vi "SegmentAndCircleIntersection.vi"(8 "CircleRadius":dbl, 9 "CircleCenter":dbl[](array[numeric]), 10 "SegmentPointB":dbl[](array[numeric]), 11 "SegmentPointA":dbl[](array[numeric])) -> (1 "DoTheyIntersect?":bool)   [LabVIEW 2017]
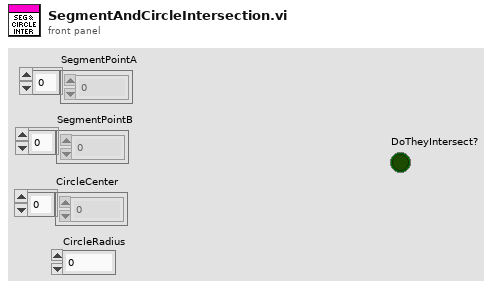
[diagram p1: front panel]
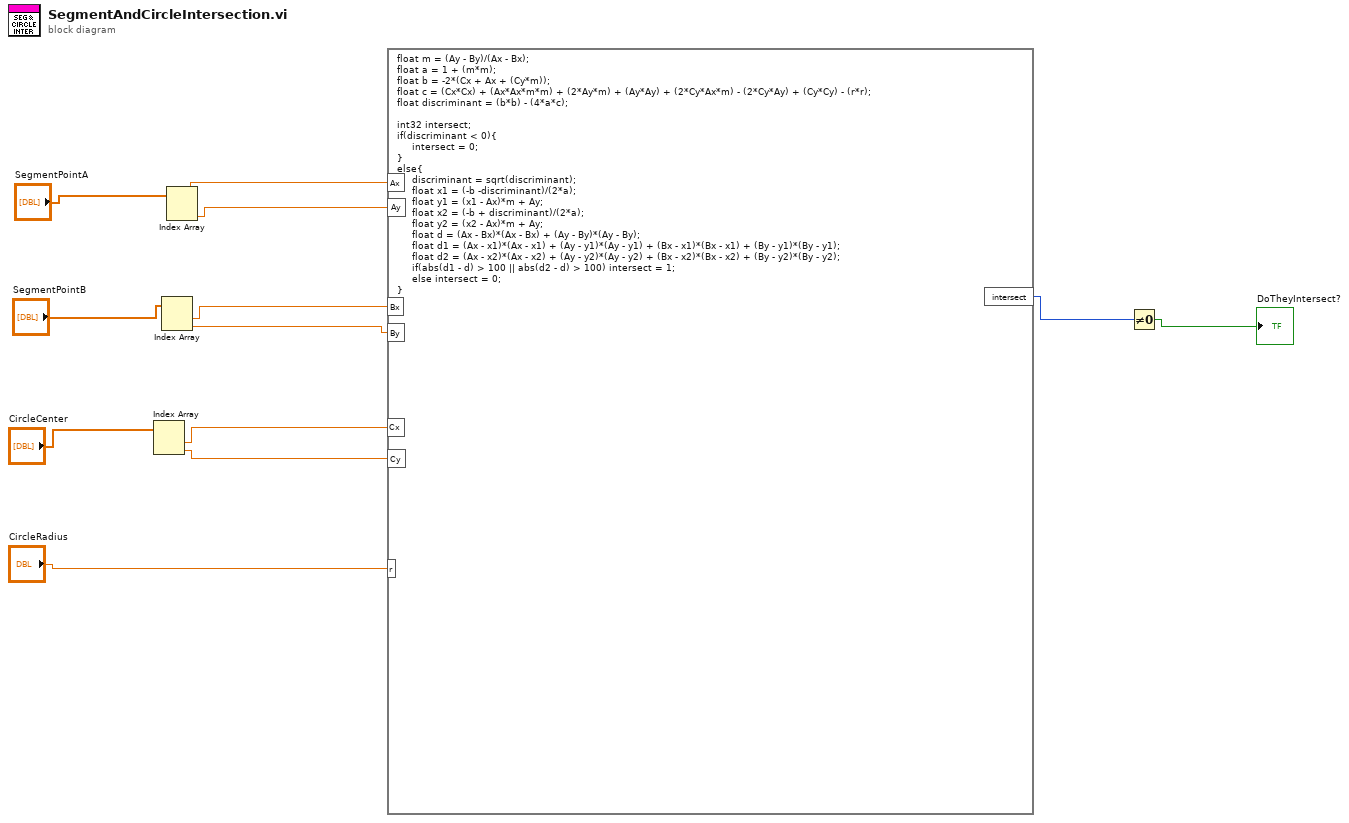
[diagram p0: block diagram]
diagram:
  n1 = Index Array(array="CircleCenter") -> (element #1=w5:dbl, element #2=w4:dbl)  [unwired: 2 in]
  n2 = Index Array(array="SegmentPointB") -> (element #1=w7:dbl, element #2=w6:dbl)  [unwired: 2 in]
  n3 = Index Array(array="SegmentPointA") -> (element #1=w8:dbl, element #2=w9:dbl)  [unwired: 2 in]
  n4 = formula code="float m = (Ay - By)/(Ax - Bx);\nfloat a = 1 + (m*m);\nfloat b = -2*(Cx + Ax + (Cy*m));\nfloat c = (Cx*Cx) + (Ax*Ax*m*m) + (2*Ay*m) + (Ay*Ay) + (2*Cy*Ax*m) - (2*Cy*Ay) + (Cy*Cy) - (r*r);\nfloat discriminant = (b*b) - (4*a*c);\n\nint32 intersect;\nif(discriminant < 0){\n     intersect = 0;\n}\nelse{\n     discriminant = sqrt(discriminant);\n     float x1 = (-b -discriminant)/(2*a);\n     float y1 = (x1 - Ax)*m + Ay;\n     float x2 = (-b + discriminant)/(2*a);\n     float y2 = (x2 - Ax)*m + Ay;\n     float d = (Ax - Bx)*(Ax - Bx) + (Ay - By)*(Ay - By);\n     float d1 = (Ax - x1)*(Ax - x1) + (Ay - y1)*(Ay - y1) + (Bx - x1)*(Bx - x1) + (By - y1)*(By - y1);\n     float d2 = (Ax - x2)*(Ax - x2) + (Ay - y2)*(Ay - y2) + (Bx - x2)*(Bx - x2) + (By - y2)*(By - y2);\n     if(abs(d1 - d) > 100 || abs(d2 - d) > 100) intersect = 1;\n     else intersect = 0;\n}"("Ax"=w8, "Ay"=w9, "Bx"=w7, "By"=w6, "Cx"=w5, "Cy"=w4, "r"="CircleRadius") -> ("intersect"=w2:i32)
  n5 = Not Equal To 0?(x=w2) -> (x != 0?=→"DoTheyIntersect?":bool)
